vi "XNET TCP Socket Read.vi"   [LabVIEW 2018]
doc: "Reads a number of bytes from a TCP network connection."
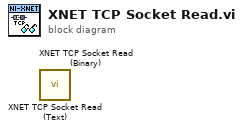
[diagram p0: block diagram]
diagram:
  n1 = call "XNET TCP Socket Read (Text).vi"() -> ()  [unwired: 9 in, 3 out]
  n2 = call "XNET TCP Socket Read (Binary).vi"() -> ()  [unwired: 9 in, 3 out]
